vi "Brenner Gradient.vi"(6 "Enum":enum16{"Reset", "Read", "Write"}(ring)=enum."Write", 11 "Live Frame":u16[][][](array[numeric])) -> (3 "Brenner Gradients":dbl[](array[numeric]))   [LabVIEW 2018]
panel:
  in  "shift length":i32=1
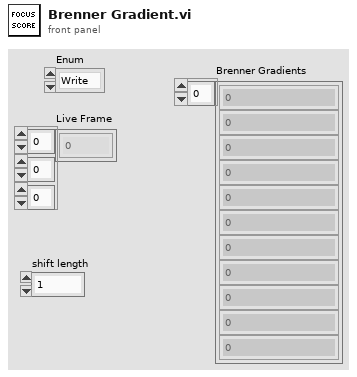
[diagram p1: front panel]
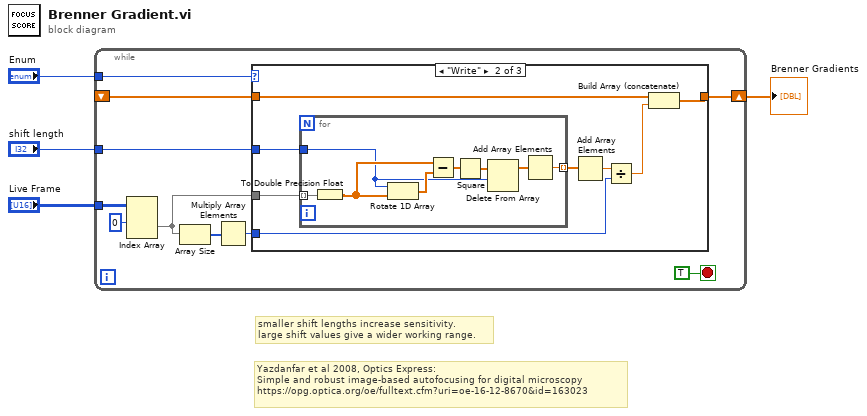
[diagram p0: block diagram]
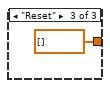
[diagram p3: hidden frame]
diagram:
  # "Yazdanfar et al 2008, Optics Express:\nSimple and robust image-based autofocusing for digital microscopy \nhttps://opg.optica.org/oe/fulltext.cfm?uri=oe-16-12-8670&id=163023"
  # "smaller shift lengths increase sensitivity.\nlarge shift values give a wider working range."
  n1 = while {
    tunnel: "shift length" -> [w14]
    shift-right: [w10] -> w3
    shift-left: _ -> [w11]
    tunnel: "Enum" -> [w8]
    tunnel: "Live Frame" -> [w6]
    stop <- TRUE stop-if-true
    n2 = Index Array(array=w6, index (dim 0)=0 ("index (page)")) -> (element=w5:u16[][])  [unwired: 2 in]
    n3 = Array Size(array=w5) -> (size(s)=w13:i32[])
    n4 = Multiply Array Elements(1:w13) -> (0:w9:i32)
    n5 = case shown="\"Write\"" w8 {
      tunnel: w5 -> [_ w23 _]
      tunnel: w14 -> [_ w22 _]
      tunnel: w11 -> [w15 w19 _]
      tunnel: [w15 w17 dbl[] []] -> w10
      tunnel: w9 -> [_ w16 _]
      frame "Read" {
      }
      frame "Write" {
        n6 = for {
          tunnel: w23 -> [w28] mode=indexing
          tunnel: [w29] -> w21 mode=indexing
          tunnel: w22 -> [w24]
          # "Loop over image rows (columns?)"
          n7 = To Double Precision Float(number=w28) -> (double precision float=w27:dbl[])
          n8 = Rotate 1D Array(1:w27, 2:w24) -> (0:w30:dbl[])
          n9 = Subtract(x=w27, y=w30) -> (x-y=w31:dbl[])
          n10 = Square(x=w31) -> (x^2=w25:dbl[])
          n11 = Delete From Array(array=w25, length=w24) -> (array with subset deleted=w26:dbl[])  [unwired: 1 in, 1 out]
          n12 = Add Array Elements(numeric array=w26) -> (sum=w29:dbl)
        }
        n13 = Add Array Elements(numeric array=w21) -> (sum=w20:dbl)
        n14 = Divide(x=w20, y=w16) -> (x/y=w18:dbl)
        n15 = Build Array (concatenate)(w19, w18) -> (w17:dbl[])
      }
      frame "Reset" {
      }
    }
  }
  "Brenner Gradients" <- w3
